vi "startServer.vi"(7 "Python path":path caption="Path to Python", 8 "error in (no error)":errorcluster, 9 "Arguments":string[](array[string]), 10 "Relative path to server file":string, 11 "LabVIEW-Python-Interface in":refnum<class "PyLVi.lvclass">) -> (0 "error out":errorcluster, 2 "standard output":string, 3 "LabVIEW-Python-Interface out":refnum<class "PyLVi.lvclass">)   [LabVIEW 2016, in "PyLVi.lvlib" / "PyLVi.lvclass"]
uses:
  PyLVi.lvclass
  PyLVi.lvclass/PyLVi.ctl
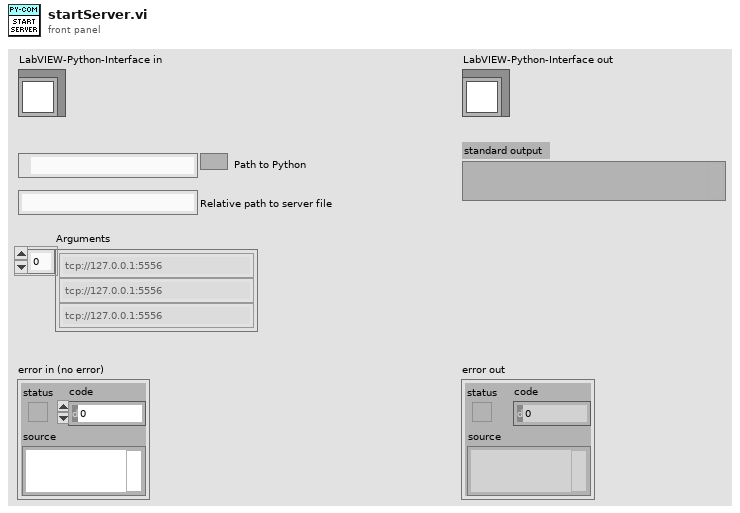
[diagram p1: front panel]
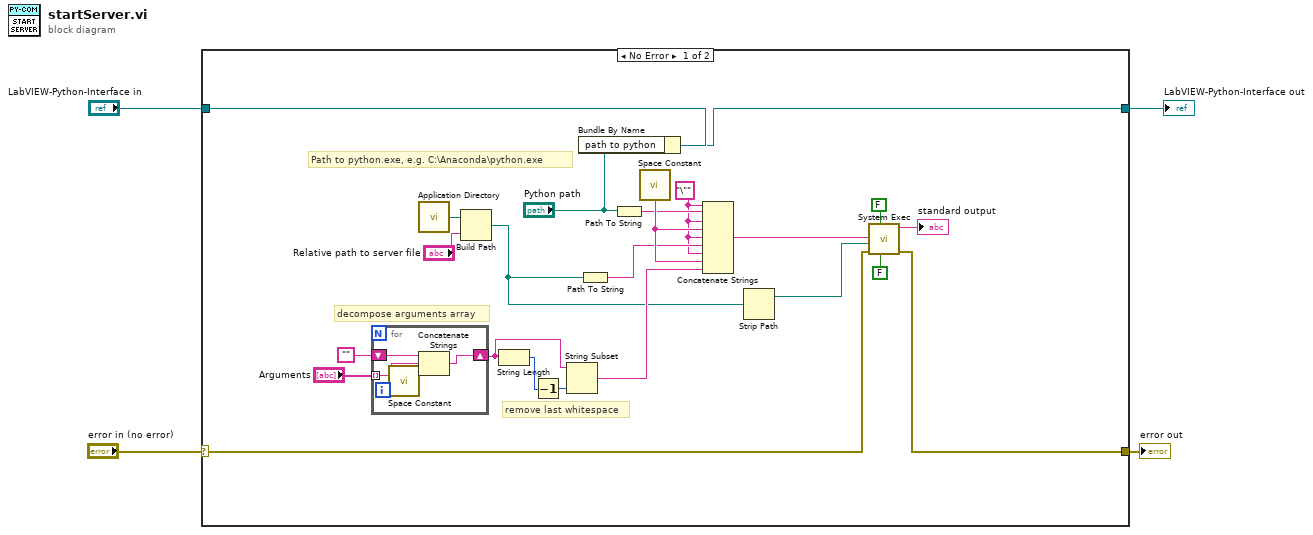
[diagram p0: block diagram]
diagram:
  n1 = case shown="No Error" "error in (no error)" {
    selector: "error in (no error)" -> [w13 w33]
    tunnel: [w12 w33] -> w3
    tunnel: [w7 w32] -> w1
    tunnel: "LabVIEW-Python-Interface in" -> [w8 w32]
    frame No Error {
      w5 = "\""
      # "remove last whitespace"
      # "decompose arguments array"
      # "Path to python.exe, e.g. C:\\Anaconda\\python.exe"
      n2 = for {
        tunnel: "Arguments" -> [w30] mode=indexing
        shift-right: [w29] -> w25
        shift-left: "" -> [w31]
        n3 = call <vilib>:"Space Constant.vi"() -> ("String"=w28:string)
        n4 = Concatenate Strings(w31, w30, w28) -> (w29:string)
      }
      n5 = call <vilib>:"Application Directory.vi"() -> ("Application Directory"=w9:path)
      n6 = Build Path(base path=w9, name or relative path="Relative path to server file") -> (appended path=w10:path)
      n7 = String Length(string=w25) -> (length=w23:i32)
      n8 = Decrement(x=w23) -> (x-1=w24:i32)
      n9 = String Subset(string=w25, length (rest)=w24) -> (substring=w26:string)  [unwired: 1 in]
      n10 = Bundle By Name(cluster=w8, "path to python"="Python path") -> (w7:refnum<class "PyLVi.lvclass">)
      n11 = Path To String(path=w10) -> (string=w19:string)
      n12 = Path To String(path="Python path") -> (string=w17:string)
      n13 = call <vilib>:"Space Constant.vi"() -> ("String"=w20:string)
      n14 = Concatenate Strings(w5, w17, w5, w20, w5, w19, w5, w20, w26) -> (w18:string)
      n15 = Strip Path(path=w10) -> (stripped path=w27:path)  [unwired: 1 out]
      n16 = call <vilib>:"System Exec.vi"("run minimized? (F)"=FALSE, "wait until completion? (T)"=FALSE, "error in (no error)"=w13, "working directory"=w27, "command line"=w18) -> ("error out"=w12:errorcluster, "standard output"=→"standard output":string)  [unwired: 3 in, 2 out]
    }
    frame Error {
    }
  }
  "error out" <- w3
  "LabVIEW-Python-Interface out" <- w1
